vi "PH_gentec_M-Link.PC get and set current Settings for the first Time - 2.vi"(0 "i ref in":refnum<vi>, 2 "VISA resource in":refnum<visa-resource-name>, 3 "Default Head Settings":T1 {"Waveform Averages" items=["None", "2", "4", "8", "16", "32", "64", "128"]; "Trigger Source" items=["Internal", "External"]; "Trigger Polarity" items=["Falling Edge", "Rising Edge"]; "Range" items=["1f", "3f", "10f", "30f", "100f", "300f", "1p", "3p", "10p", "30p", "100p", "300p", "1n", "3n", "10n", "30n", "100n", "300n", "1u", "3u", "10u", "30u", "100u", "300u", "1m", "3m", "10m", "30m", "100m", "300m", "1", "3", "10", "30", "100", "300", "1K", "3K", "10K", "30K", "100K", "300K", "1M", "3M", "10M", "30M", "100M", "300M"]; "Measurement Mode" items=["other Mode", "Energymode"]}, 5 "error in":errorcluster) -> (14 "i ref out":refnum<vi>, 16 "VISA resource out":refnum<visa-resource-name>, 19 "error out":errorcluster)   [LabVIEW 2009, in "PH_gentec_M-Link.lvlib"]
doc: "This VI gets and sets all current settings for the first time."
uses:
  PH_gentec_M-Link.lvlib
  PH_gentec_M-Link.Head Settings.ctl
  non_GPL/instr.lib/gentec-M-LINK/Driver/Type Defs/gentec-M-Link.Measurement Mode.ctl
  non_GPL/instr.lib/gentec-M-LINK/Driver/Type Defs/gentec-M-Link.Range.ctl
  non_GPL/instr.lib/gentec-M-LINK/Driver/Type Defs/gentec-M-Link.Trigger Polarity.ctl
  non_GPL/instr.lib/gentec-M-LINK/Driver/Type Defs/gentec-M-Link.Trigger Source.ctl
  non_GPL/instr.lib/gentec-M-LINK/Driver/Type Defs/gentec-M-Link.Waveform Averages.ctl
  non_GPL/instr.lib/gentec-M-LINK/Driver/Type Defs/gentec-M-Link.Range Queries.ctl
  non_GPL/instr.lib/gentec-M-LINK/gentec-M-LINK.lvlib
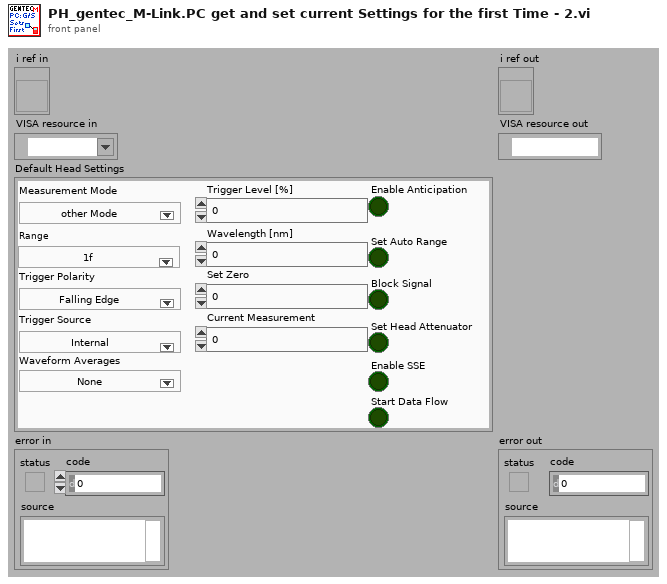
[diagram p1: front panel]
types:
  T1 = typedef "PH_gentec_M-Link.lvlib/PH_gentec_M-Link.Head Settings.ctl" = cluster{"Measurement Mode":T2, "Enable Anticipation":bool, "Set Auto Range":bool, "Block Signal":bool, "Set Head Attenuator":bool, "Range":T3, "Enable SSE":bool, "Trigger Level [%]":dbl, "Trigger Polarity":T4, "Trigger Source":T5, "Waveform Averages":T6, "Wavelength [nm]":u16, "Set Zero":i32, "Current Measurement":i32, "Start Data Flow":bool}
  T2 = typedef "gentec-M-LINK.lvlib/gentec-M-Link.Measurement Mode.ctl" = u16
  T3 = typedef "gentec-M-LINK.lvlib/gentec-M-Link.Range.ctl" = u16
  T4 = typedef "gentec-M-LINK.lvlib/gentec-M-Link.Trigger Polarity.ctl" = u16
  T5 = typedef "gentec-M-LINK.lvlib/gentec-M-Link.Trigger Source.ctl" = u16
  T6 = typedef "gentec-M-LINK.lvlib/gentec-M-Link.Waveform Averages.ctl" = u16
  T7 = typedef "PH_gentec_M-Link.lvlib/PH_gentec_M-Link.i attribute.ctl" = cluster{"GUI References":cluster{"Status":refnum<vi>, "Status Bar":refnum<vi>, "Head Attributes":refnum<vi>, "Wanted Head Settings":refnum<vi>, "Current Head Settings":refnum<vi>, "unscaled Energy [J]":refnum<vi>, "Energy [J]":refnum<vi>, "Energy evolution":refnum<vi>, "Set Auto Range":refnum<vi>, "Range":refnum<vi>, "Trigger Level [%]":refnum<vi>, "Trigger Polarity":refnum<vi>, "Trigger Source":refnum<vi>, "Waveform Averages":refnum<vi>, "Wavelength [nm]":refnum<vi>, "Continuous":refnum<vi>, "Scaling Factor":refnum<vi>, "Connection":refnum<vi>, "Sets 2 change?":refnum<vi>, "get one Value":refnum<vi>}, "Constructor finished?":bool, "GUI Manager Path":string, "Connection":T8, "Head Attributes":T9, "Wanted Head Settings":T1, "Current Head Settings":T1, "Scaling Factor":dbl, "Energy [J]":dbl, "Settings to change?":bool}
  T8 = typedef "PH_gentec_M-Link.lvlib/PH_gentec_M-Link.Connection.ctl" = cluster{"opened":bool, "checked":bool, "failed checks":i8, "Info available":bool, "Timeout":bool, "Data read":string, "Failure":bool, "Error":bool}
  T9 = typedef "PH_gentec_M-Link.lvlib/PH_gentec_M-Link.Head Attributes.ctl" = cluster{"Instrument Type":string, "Head Version":string, "Head Name":string, "Serial Number":string, "Firmware":string, "Sensor Type":T10, "Minimum Range":T3, "Maximum Range":T3, "Minimum Lambda [nm]":i32, "Maximum Lambda [nm]":i32}
  T10 = typedef "gentec-M-LINK.lvlib/gentec-M-Link.Sensor Type.ctl" = u16
  T11 = typedef "gentec-M-LINK.lvlib/gentec-M-Link.Range Queries.ctl" = string
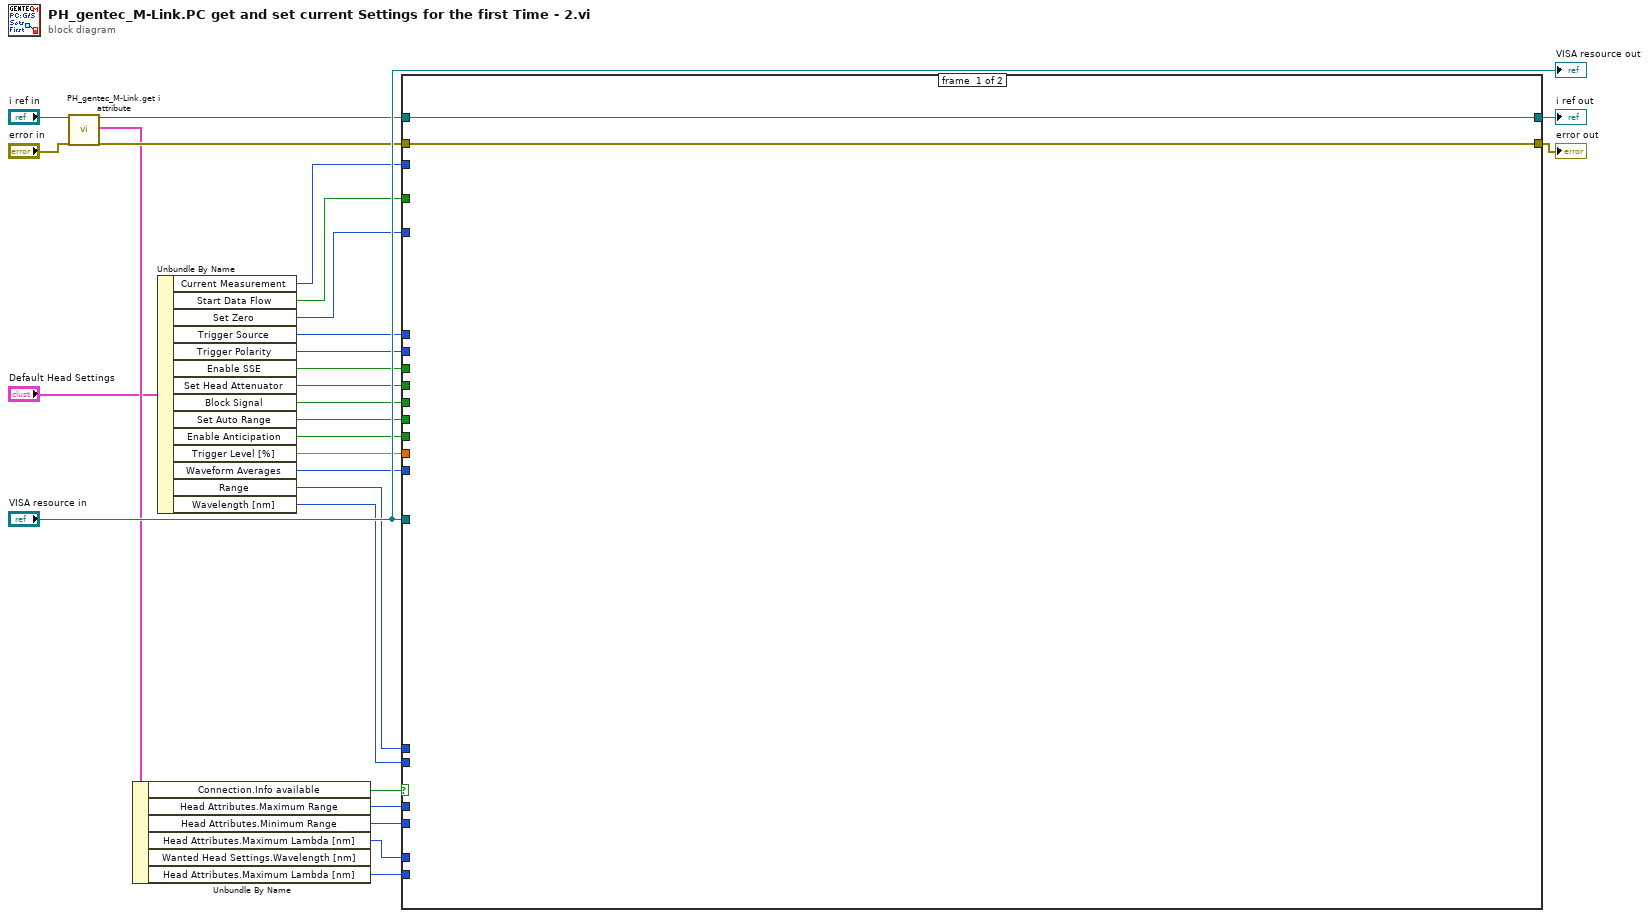
[diagram p0: block diagram]
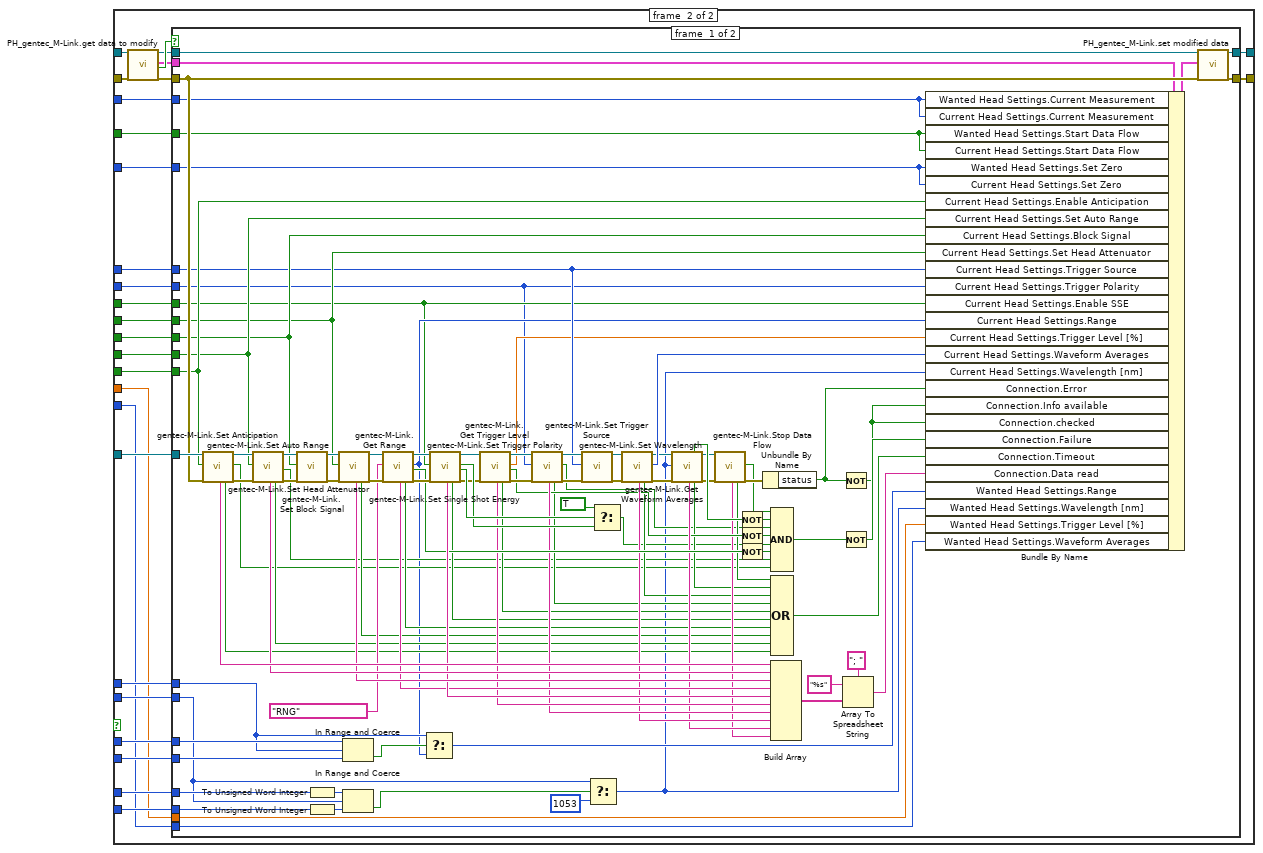
[diagram p2: hidden frame]
diagram:
  n1 = call "PH_gentec_M-Link.get i attribute.vi"("i ref in"="i ref in", "error in (no error)"="error in") -> ("i ref out"=w24:refnum<vi>, "i attribute"=w21:T7, "error out"=w22:errorcluster)  [unwired: 15 in]
  n2 = Unbundle By Name(w21) -> ("Connection.Info available"=w20:bool, "Head Attributes.Maximum Range"=w19:T3, "Head Attributes.Minimum Range"=w18:T3, "Head Attributes.Maximum Lambda [nm]"=w17:i32, "Head Attributes.Maximum Lambda [nm]"=w16:i32)  [unwired: 1 out]
  n3 = Unbundle By Name("Default Head Settings") -> ("Current Measurement"=w3:i32, "Start Data Flow"=w2:bool, "Set Zero"=w1:i32, "Trigger Source"=w6:T5, "Trigger Polarity"=w7:T4, "Enable SSE"=w10:bool, "Set Head Attenuator"=w11:bool, "Block Signal"=w12:bool, "Set Auto Range"=w13:bool, "Enable Anticipation"=w14:bool, "Trigger Level [%]"=w8:dbl, "Waveform Averages"=w5:T6, "Range"=w9:T3, "Wavelength [nm]"=w4:u16)
  n4 = case shown="True" w20 {
    tunnel: [w29 w53] -> w28
    tunnel: [w30 w52] -> w27
    tunnel: "VISA resource in" -> [_ w51]
    tunnel: w24 -> [w30 w50]
    tunnel: w22 -> [w29 w49]
    tunnel: w9 -> [_ w48]
    tunnel: w19 -> [_ w47]
    tunnel: w18 -> [_ w46]
    tunnel: w17 -> [_ w45]
    tunnel: w4 -> [_ w44]
    tunnel: w16 -> [_ w43]
    tunnel: w14 -> [_ w42]
    tunnel: w13 -> [_ w41]
    tunnel: w12 -> [_ w40]
    tunnel: w11 -> [_ w39]
    tunnel: w10 -> [_ w38]
    tunnel: w8 -> [_ w37]
    tunnel: w7 -> [_ w36]
    tunnel: w6 -> [_ w35]
    tunnel: w5 -> [_ w34]
    tunnel: w3 -> [_ w33]
    tunnel: w2 -> [_ w32]
    tunnel: w1 -> [_ w31]
    frame #0 {
    }
    frame #1 {
      n5 = call "PH_gentec_M-Link.get data to modify.vi"("i ref in"=w50, "error in (no error)"=w49) -> ("i ref out"=w55:refnum<vi>, "i attribute"=w56:T7, "timed out"=w57:bool, "error out"=w54:errorcluster)  [unwired: 14 in]
      n6 = case shown="False" w57 {
        tunnel: w51 -> [w156 _]
        tunnel: [w159 w161] -> w52
        tunnel: [w158 w160] -> w53
        tunnel: w54 -> [w153 w160]
        tunnel: w55 -> [w157 w161]
        tunnel: w56 -> [w138 _]
        tunnel: w48 -> [w77 _]
        tunnel: w47 -> [w84 _]
        tunnel: w46 -> [w83 _]
        tunnel: w45 -> [w82 _]
        tunnel: w44 -> [w74 _]
        tunnel: w43 -> [w81 _]
        tunnel: w42 -> [w73 _]
        tunnel: w41 -> [w72 _]
        tunnel: w40 -> [w71 _]
        tunnel: w39 -> [w70 _]
        tunnel: w38 -> [w62 _]
        tunnel: w37 -> [w69 _]
        tunnel: w36 -> [w61 _]
        tunnel: w35 -> [w68 _]
        tunnel: w34 -> [w67 _]
        tunnel: w33 -> [w60 _]
        tunnel: w32 -> [w59 _]
        tunnel: w31 -> [w58 _]
        frame #0 {
          n7 = call "gentec-M-Link.Set Anticipation.vi"("VISA resource In"=w156, "Enable Anticipation"=w73, "error in (no error)"=w153) -> ("Data Read"=w148:string, "Read Timeout"=w95:bool, "VISA resource Out"=w154:refnum<visa-resource-name>, "Success"=w86:bool, "error out"=w152:errorcluster)  [unwired: 12 in]
          n8 = call "gentec-M-Link.Set Auto Range.vi"("VISA resource In"=w154, "Auto Range"=w72, "error in (no error)"=w152) -> ("Data Read"=w147:string, "Read Timeout"=w96:bool, "VISA resource Out"=w155:refnum<visa-resource-name>, "Success"=w87:bool, "error out"=w151:errorcluster)  [unwired: 12 in]
          n9 = call "gentec-M-Link.Set Block Signal.vi"("VISA resource In"=w155, "Block Signal"=w71, "error in (no error)"=w151) -> ("VISA resource Out"=w150:refnum<visa-resource-name>, "error out"=w149:errorcluster)  [unwired: 15 in]
          n10 = To Unsigned Word Integer(number=w82) -> (unsigned 16bit integer=w80:u16)
          n11 = To Unsigned Word Integer(number=w81) -> (unsigned 16bit integer=w79:u16)
          n12 = call "gentec-M-Link.Set Head Attenuator.vi"("VISA resource In"=w150, "Set Head Attenuator"=w70, "error in (no error)"=w149) -> ("Data Read"=w146:string, "Read Timeout"=w97:bool, "VISA resource Out"=w133:refnum<visa-resource-name>, "error out"=w131:errorcluster)  [unwired: 11 in, 2 out]
          n13 = In Range and Coerce(upper limit=w84, x=w77, lower limit=w83) -> (In Range?=w78:bool)  [unwired: 1 out]
          n14 = In Range and Coerce(upper limit=w80, x=w74, lower limit=w79) -> (In Range?=w75:bool)  [unwired: 1 out]
          n15 = call "gentec-M-Link.Get Range.vi"("VISA resource In"=w133, "Range Queries"=T11 "RNG", "error in (no error)"=w131) -> ("Data Read"=w128:string, "Read Timeout"=w98:bool, "VISA resource Out"=w132:refnum<visa-resource-name>, "Range"=w63:T3, "Error"=w127:bool, "error out"=w130:errorcluster)  [unwired: 11 in]
          n16 = Select(t=w77, s=w78, f=w63) -> (s? t:f=w76:T3)
          n17 = call "gentec-M-Link.Set Single Shot Energy.vi"("VISA resource In"=w132, "Enable Single Shot Energy"=w62, "error in (no error)"=w130) -> ("Data Read"=w145:string, "Read Timeout"=w99:bool, "VISA resource Out"=w126:refnum<visa-resource-name>, "Success"=w140:bool, "no Thermopyle Head"=w141:bool, "error out"=w125:errorcluster)  [unwired: 11 in]
          n18 = call "gentec-M-Link.Get Trigger Level.vi"("VISA resource In"=w126, "error in (no error)"=w125) -> ("Data Read"=w124:string, "Read Timeout"=w100:bool, "VISA resource Out"=w121:refnum<visa-resource-name>, "Trigger Level [%]"=w64:dbl, "Error"=w110:bool, "error out"=w123:errorcluster)  [unwired: 12 in]
          n19 = call "gentec-M-Link.Set Trigger Polarity.vi"("VISA resource In"=w121, "Trigger Polarity"=w61, "error in (no error)"=w123) -> ("Data Read"=w119:string, "Read Timeout"=w101:bool, "VISA resource Out"=w120:refnum<visa-resource-name>, "Success"=w91:bool, "error out"=w122:errorcluster)  [unwired: 12 in]
          n20 = call "gentec-M-Link.Set Trigger Source.vi"("VISA resource In"=w120, "Trigger Source"=w68, "error in (no error)"=w122) -> ("VISA resource Out"=w118:refnum<visa-resource-name>, "error out"=w117:errorcluster)  [unwired: 15 in]
          n21 = Select(t=w74, s=w75, f=u16 1053) -> (s? t:f=w65:u16)
          n22 = Select(t=TRUE, s=w141, f=w140) -> (s? t:f=w89:bool)
          n23 = call "gentec-M-Link.Get Waveform Averages.vi"("VISA resource In"=w118, "error in (no error)"=w117) -> ("Data Read"=w116:string, "Read Timeout"=w102:bool, "VISA resource Out"=w113:refnum<visa-resource-name>, "Waveform Averages"=w115:T6, "error out"=w114:errorcluster)  [unwired: 13 in]
          n24 = call "gentec-M-Link.Set Wavelength.vi"("VISA resource In"=w113, "Lambda"=w65, "error in (no error)"=w114) -> ("Data Read"=w112:string, "Error"=w111:bool, "Read Timeout"=w103:bool, "VISA resource Out"=w107:refnum<visa-resource-name>, "error out"=w109:errorcluster)  [unwired: 8 in, 4 out]
          n25 = call "gentec-M-Link.Stop Data Flow.vi"("VISA resource In"=w107, "error in (no error)"=w109) -> ("Data Read"=w105:string, "Read Timeout"=w104:bool, "Success"=w93:bool, "error out"=w108:errorcluster)  [unwired: 13 in, 1 out]
          n26 = Not(x=w111) -> (.not. x?=w92:bool)
          n27 = Not(x=w110) -> (.not. x?=w90:bool)
          n28 = Not(x=w127) -> (.not. x?=w88:bool)
          n29 = Unbundle By Name(w108) -> ("status"=w135:bool)
          n30 = Compound Arithmetic op=AND(w93, w92, w91, w90, w89, w88, w87, w86) -> (w85:bool)
          n31 = Compound Arithmetic op=OR(w104, w103, w102, w101, w100, w99, w98, w97, w96, w95) -> (w94:bool)
          n32 = Build Array(w148, w147, w146, w128, w145, w124, w119, w116, w112, w105) -> (w142:string[])
          n33 = Not(x=w135) -> (.not. x?=w106:bool)
          n34 = Not(x=w85) -> (.not. x?=w136:bool)
          n35 = Array To Spreadsheet String(delimiter (Tab)="; ", array=w142, 3:"%s" ("format string")) -> (spreadsheet string=w137:string)
          n36 = Bundle By Name(cluster=w138, "Wanted Head Settings.Current Measurement"=w60, "Current Head Settings.Current Measurement"=w60, "Wanted Head Settings.Start Data Flow"=w59, "Current Head Settings.Start Data Flow"=w59, "Wanted Head Settings.Set Zero"=w58, "Current Head Settings.Set Zero"=w58, "Current Head Settings.Enable Anticipation"=w73, "Current Head Settings.Set Auto Range"=w72, "Current Head Settings.Block Signal"=w71, "Current Head Settings.Set Head Attenuator"=w70, "Current Head Settings.Trigger Source"=w68, "Current Head Settings.Trigger Polarity"=w61, "Current Head Settings.Enable SSE"=w62, "Current Head Settings.Range"=w63, "Current Head Settings.Trigger Level [%]"=w64, "Current Head Settings.Waveform Averages"=w115, "Current Head Settings.Wavelength [nm]"=w65, "Connection.Error"=w135, "Connection.Info available"=w106, "Connection.checked"=w106, "Connection.Failure"=w136, "Connection.Timeout"=w94, "Connection.Data read"=w137, "Wanted Head Settings.Range"=w76, "Wanted Head Settings.Wavelength [nm]"=w65, "Wanted Head Settings.Trigger Level [%]"=w69, "Wanted Head Settings.Waveform Averages"=w67) -> (w134:T7)
          n37 = call "PH_gentec_M-Link.set modified data.vi"("i ref in"=w157, "i attribute"=w134, "error in (no error)"=w153) -> ("i ref out"=w159:refnum<vi>, "error out"=w158:errorcluster)  [unwired: 15 in]
        }
        frame #1 {
        }
      }
    }
  }
  "error out" <- w28
  "i ref out" <- w27
  "VISA resource out" <- "VISA resource in"
